vi "Read File.vi"(11 "Game Board in":refnum<class "Game Board.lvclass">) -> (0 "error out":errorcluster, 3 "Game Board out":refnum<class "Game Board.lvclass">)   [LabVIEW 2021, in "Game Board.lvclass"]
doc: "MIT Licence\nCopyright (c) 2024 David Grollier"
uses:
  Game Board.lvclass
  Game Board Component/Movable/Movable.lvclass
  C:/Users/David/Documents/GameSoccerSpace/Source/Game Componants/Game Board Component/Game Board Component.lvclass
  Game Board.lvclass/Game Board.ctl
  Game Board Component/Game Board Component.lvclass/Game Board Component.ctl
  Game Board Component/Game Board Component.lvclass
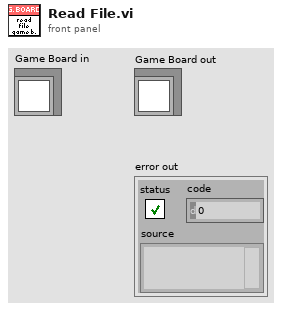
[diagram p1: front panel]
types:
  T1 = map{string, refnum<class "Game Board Component.lvclass">}
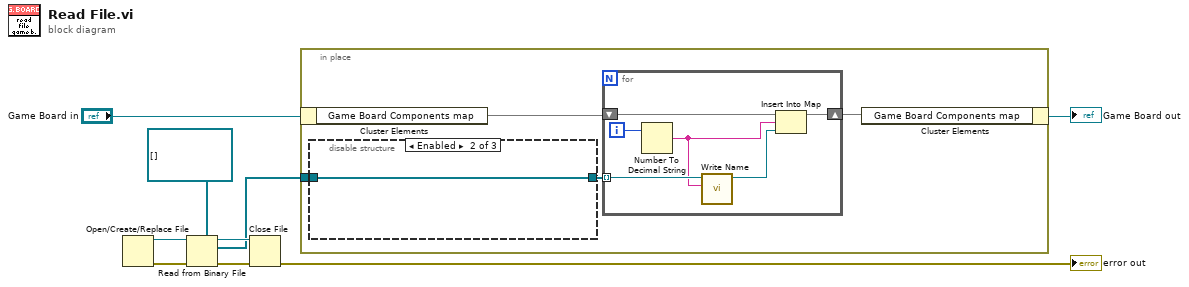
[diagram p0: block diagram]
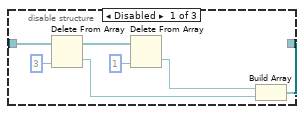
[diagram p2: hidden frame]
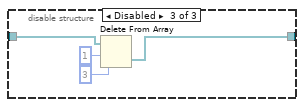
[diagram p3: hidden frame]
diagram:
  n1 = Open/Create/Replace File() -> (refnum out=w9:refnum<file>, error out=w5:errorcluster)  [unwired: 6 in, 1 out]
  n2 = Read from Binary File(5:refnum<class "Movable.lvclass">[] [], 8:w5, 11:w9) -> (0:w7:errorcluster, 2:w3:refnum<class "Movable.lvclass">[], 3:w8:refnum<file>)  [unwired: 3 in, 1 out]
  n3 = Close File(refnum=w8, error in=w7) -> (error out=→"error out":errorcluster)  [unwired: 1 out]
  n4 = in-place {
    in-place-border: w3 -> [w13]
    n5 = in-place-cluster #1("Game Board in") -> ("Game Board Components map"=w12:T1)
    n6 = disable-structure shown="Enabled" {
      disable-tunnel: w13 -> [w20 w21 w25]
      disable-tunnel: [w16 w21 w23] -> w10
      frame Disabled {
        n7 = Delete From Array(array=w20, index=3) -> (deleted portion=w17:refnum<class "Movable.lvclass">, array with subset deleted=w19:refnum<class "Movable.lvclass">[])  [unwired: 1 in]
        n8 = Delete From Array(array=w19, index=1) -> (deleted portion=w14:refnum<class "Movable.lvclass">)  [unwired: 1 in, 1 out]
        n9 = Build Array(w14, w17) -> (w16:refnum<class "Movable.lvclass">[])
      }
      frame Enabled {
      }
      frame Disabled {
        n10 = Delete From Array(array=w25, length=1, index=3) -> (deleted portion=w23:refnum<class "Movable.lvclass">[])  [unwired: 1 out]
      }
    }
    n11 = for {
      shift-right: [w30] -> w11
      shift-left: w12 -> [w31]
      tunnel: w10 -> [w28] mode=indexing
      i -> [w29]
      n12 = Number To Decimal String(number=w29) -> (decimal integer string=w27:string)  [unwired: 1 in]
      n13 = call "Write Name.vi"("Name"=w27, "Game Board Component in"=w28) -> ("Game Board Component out"=w26:refnum<class "Movable.lvclass">)  [unwired: 9 in]
      n14 = Insert Into Map(map in=w31, key=w27, value=w26) -> (map out=w30:T1)  [unwired: 2 out]
    }
    n15 = in-place-cluster #1("Game Board Components map"=w11) -> (→"Game Board out":refnum<class "Game Board.lvclass">)
  }
